vi "Find All Instruments.vi"() -> (0 "error out (no error)":errorcluster, 1 "Cancel Out":bool, 2 "List of Instruments Out":T1[](array[typedef]))   [LabVIEW 2013, in "SetUp VIs.lvlib"]
uses:
  SetUp VIs.lvlib
  Controls/Instrument ID Object.ctl
panel:
  in  "Cancle":bool
  in  "Done":bool
  out "# of Instruments Found":i32
  in  "List of Instruments":T1[](array[typedef])
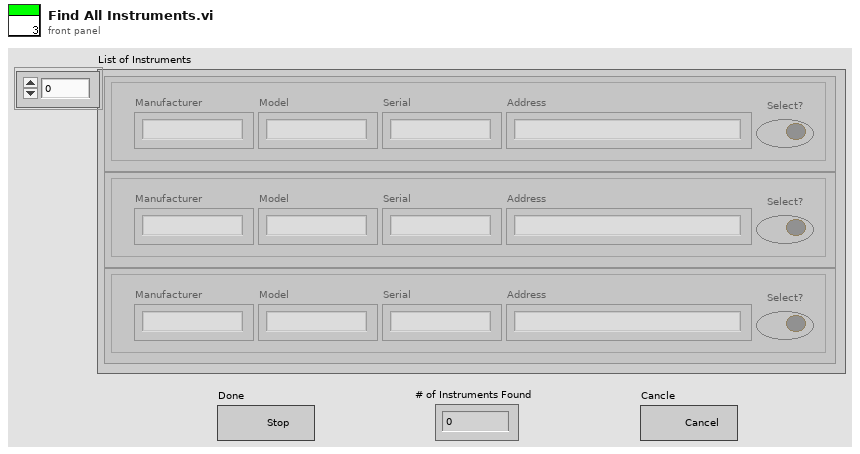
[diagram p1: front panel]
types:
  T1 = typedef "Instrument ID Object.ctl" = cluster{"Manufacturer":string, "Model":string, "Serial":string, "Address":string, "Select?":bool}
  T2 = cluster{"Manufacturer":string, "Model":string, "Serial":string, "Address":string, bool}
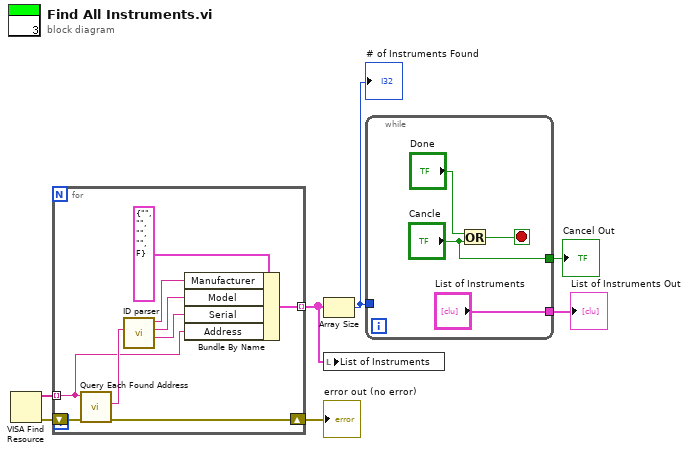
[diagram p0: block diagram]
diagram:
  n1 = VISA Find Resource() -> (0:w5:errorcluster, 3:w7:string[])  [unwired: 3 in, 1 out]
  n2 = for {
    tunnel: w7 -> [w14] mode=indexing
    tunnel: [w10] -> w4 mode=indexing
    shift-right: [w9] -> w6
    shift-left: w5 -> [w8]
    n3 = call "Query Each Found Address.vi"("error in (no error) 2"=w8, "Address"=w14) -> ("error out (no error)"=w9:errorcluster, "read buffer"=w16:string)  [unwired: 8 in]
    n4 = call "ID parser.vi"("Input String"=w16) -> ("Serial"=w11:string, "Model"=w12:string, "Manufacturer"=w13:string)  [unwired: 8 in]
    n5 = Bundle By Name(cluster=T2 {"Manufacturer"="", "Model"="", "Serial"="", "Address"="", FALSE} ("Instrument"), "Manufacturer"=w13, "Model"=w12, "Serial"=w11, "Address"=w14) -> (w10:T2)
  }
  "error out (no error)" <- w6
  n6 = Array Size(array=w4) -> (size(s)=w3:i32)
  "# of Instruments Found" <- w3
  n7 = local write "List of Instruments"(w4) -> ()
  n8 = while {
    tunnel: w3 -> [_]
    tunnel: ["List of Instruments"] -> w2
    tunnel: ["Cancle"] -> w1
    stop <- w18 stop-if-true
    n9 = Or(x="Done", y="Cancle") -> (x .or. y?=w18:bool)
  }
  "List of Instruments Out" <- w2
  "Cancel Out" <- w1
